vi "VDH-createDataFile.vi"(7 "file path (use dialog)":path, 8 "error in (no error)":errorcluster, 10 "Data":T1, 11 "VDH-VNA_data_handler in":refnum<class "VDH-VNA_data_handler.lvclass">) -> (0 "error out":errorcluster, 3 "VDH-VNA_data_handler out":refnum<class "VDH-VNA_data_handler.lvclass">)   [LabVIEW 2020, in "VDH-VNA_data_handler.lvlib" / "VDH-VNA_data_handler.lvclass"]
uses:
  VDH-VNA_data_handler.lvclass
  VDH-VNA_data.ctl
  <vilib>/Utility/file.llb/Write Delimited Spreadsheet (DBL).vi
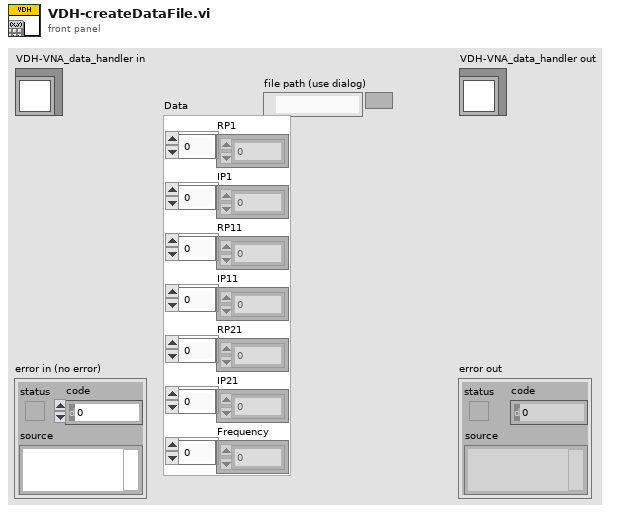
[diagram p1: front panel]
types:
  T1 = typedef "VDH-VNA_data_handler.lvlib/VDH-VNA_data_handler.lvclass/VDH-VNA_data.ctl" = cluster{"RP1":dbl[], "IP1":dbl[], "RP11":dbl[], "IP11":dbl[], "RP21":dbl[], "IP21":dbl[], "Frequency":u64[]}
  T2 = enum16{"open", "replace", "create", "open or create", "replace or create", "replace or create with confirmation"}
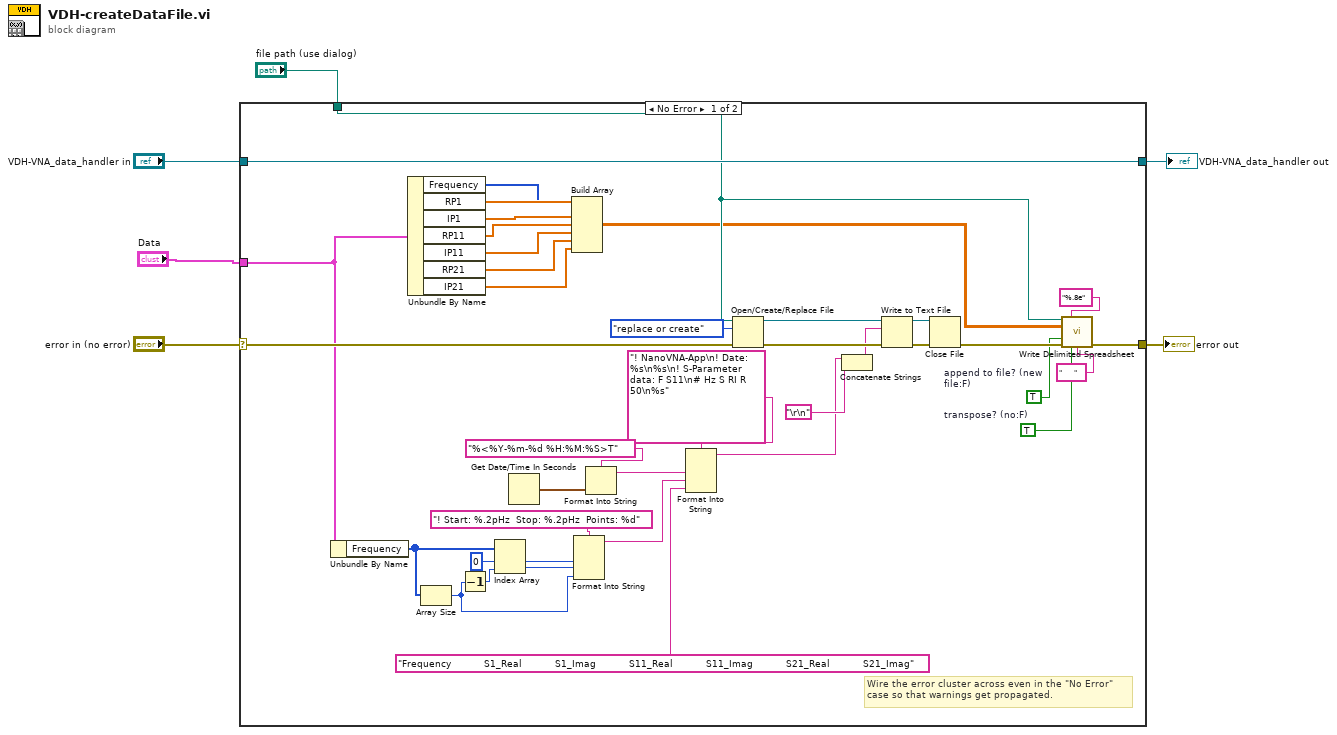
[diagram p0: block diagram]
diagram:
  n1 = case shown="No Error" "error in (no error)" {
    selector: "error in (no error)" -> [w15 w47]
    tunnel: [w7 w47] -> w5
    tunnel: [w26 w46] -> w3
    tunnel: "VDH-VNA_data_handler in" -> [w26 w46]
    tunnel: "Data" -> [w8 _]
    tunnel: "file path (use dialog)" -> [w24 _]
    frame No Error {
      w27 = TRUE  # append to file? (new file:F)
      w29 = TRUE  # transpose? (no:F)
      # "Wire the error cluster across even in the \"No Error\"\ncase so that warnings get propagated."
      n2 = Unbundle By Name(w8) -> ("Frequency"=w14:u64[])
      n3 = Unbundle By Name(w8) -> ("Frequency"=w21:u64[], "RP1"=w23:dbl[], "IP1"=w22:dbl[], "RP11"=w20:dbl[], "IP11"=w19:dbl[], "RP21"=w18:dbl[], "IP21"=w17:dbl[])
      n4 = Array Size(array=w14) -> (size(s)=w9:i32)
      n5 = Decrement(x=w9) -> (x-1=w13:i32)
      n6 = Index Array(array=w14, index #1=0 ("index"), index #2=w13) -> (element #1=w11:u64, element #2=w10:u64)
      n7 = Get Date/Time In Seconds() -> (seconds since 1Jan1904=w36:timestamp)
      n8 = Build Array(w21, w23, w22, w20, w19, w18, w17) -> (w16:dbl[][])
      n9 = Format Into String(format string="! Start: %.2pHz  Stop: %.2pHz  Points: %d", w11, w10, w9) -> (resulting string=w32:string)  [unwired: 2 in, 1 out]
      n10 = Format Into String(format string="%<%Y-%m-%d %H:%M:%S>T", w36) -> (resulting string=w34:string)  [unwired: 2 in, 1 out]
      n11 = Format Into String(format string="! NanoVNA-App\n! Date: %s\n%s\n! S-Parameter data: F S11\n# Hz S RI R 50\n%s" ("text"), w34, w32, "Frequency           S1_Real           S1_Imag           S11_Real           S11_Imag           S21_Real           S21_Imag" ("input 3")) -> (resulting string=w38:string)  [unwired: 2 in, 1 out]
      n12 = Open/Create/Replace File(file path (use dialog)=w24, error in=w15, operation (0:open)=T2."replace or create") -> (refnum out=w42:refnum<file>, error out=w43:errorcluster)  [unwired: 3 in, 1 out]
      n13 = Concatenate Strings(w38, "\r\n") -> (w39:string)
      n14 = Write to Text File(file (use dialog)=w42, text=w39, error in=w43) -> (refnum out=w44:refnum<file>, error out=w45:errorcluster)  [unwired: 1 in, 1 out]
      n15 = Close File(refnum=w44, error in=w45) -> (error out=w28:errorcluster)  [unwired: 1 out]
      n16 = call-poly <vilib>:"Write Delimited Spreadsheet.vi"("file path (dialog if empty)"=w24, "format (%.3f)"="%.8e", "2D data"=w16, "append to file? (new file:F)"=w27, "error in (no error)"=w28, "transpose? (no:F)"=w29, "delimiter (\\t)"="      " ("delimiter (\\t)")) -> ("error out"=w7:errorcluster)  [unwired: 7 in, 1 out]
    }
    frame Error {
    }
  }
  "error out" <- w5
  "VDH-VNA_data_handler out" <- w3
